vi "Pacemaker Final.vi"() -> ()   [LabVIEW 2018]
panel:
  out "Filtered ECG + Pacemaker Impulses":cluster{"Y":dbl[], dbl[]}[](graph)
  in  "Spreadsheet Path (.csv)":path
  out "ECG Data":dbl[](array[numeric])
  out "Original ECG":waveform(dbl)(graph)
  out "Time Data":dbl
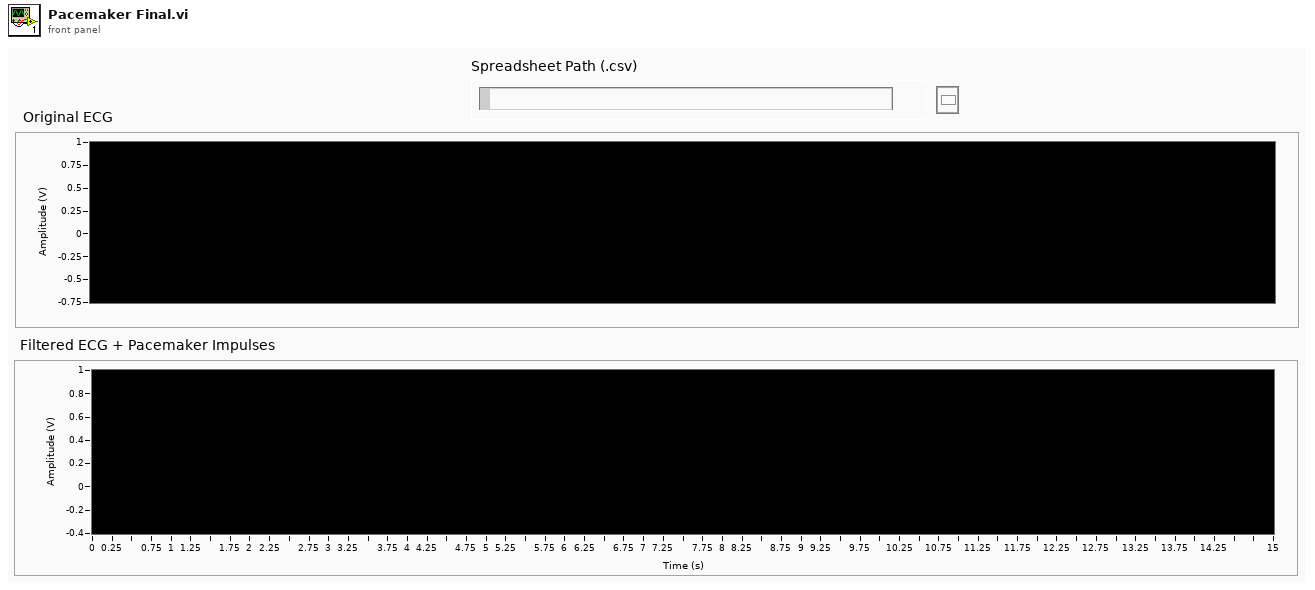
[diagram p1: front panel]
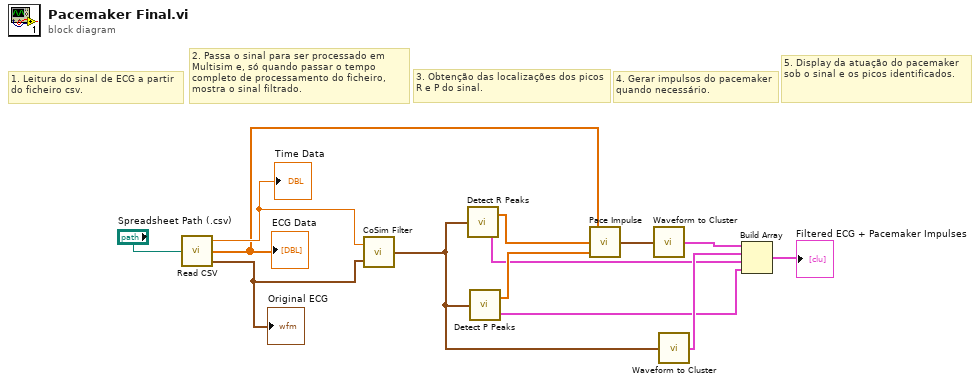
[diagram p0: block diagram]
diagram:
  # "4. Gerar impulsos do pacemaker quando necessário."
  # "3. Obtenção das localizações dos picos R e P do sinal."
  # "5. Display da atuação do pacemaker sob o sinal e os picos identificados."
  # "1. Leitura do sinal de ECG a partir do ficheiro csv."
  # "2. Passa o sinal para ser processado em Multisim e, só quando passar o tempo completo de processamento do ficheiro, mostra o sinal filtrado."
  n1 = call "Read CSV.vi"("file path (dialog if empty)"="Spreadsheet Path (.csv)") -> ("Time Data"=w12:dbl, "ECG Data"=w11:dbl[], "Original ECG"=w10:waveform(dbl))
  "ECG Data" <- w11
  "Original ECG" <- w10
  "Time Data" <- w12
  n2 = call "CoSim Filter.vi"("Original ECG"=w10, "Time Data"=w12) -> ("Filtered ECG"=w6:waveform(dbl))
  n3 = call "Detect R Peaks.vi"("Filtered ECG"=w6) -> ("R-Wave Locations (s)"=w8:dbl[], "Coordinates"=w2:cluster{dbl[], dbl[]})
  n4 = call "Detect P Peaks.vi"("Filtered ECG"=w6) -> ("P-Waves Locations (s)"=w7:dbl[], "Coordinates"=w1:cluster{dbl[], dbl[]})
  n5 = call "Pace Impulse.vi"("P-Waves Locations (s)"=w7, "R-Wave Locations (s)"=w8, "ECG Data"=w11) -> ("Impulses"=w9:waveform(dbl))
  n6 = call "Waveform to Cluster.vi"("Waveform"=w9) -> ("Clustered  Wave"=w4:cluster{"Y":dbl[], dbl[]})
  n7 = call "Waveform to Cluster.vi"("Waveform"=w6) -> ("Clustered  Wave"=w3:cluster{"Y":dbl[], dbl[]})
  n8 = Build Array(w4, w3, w2, w1) -> (→"Filtered ECG + Pacemaker Impulses":cluster{"Y":dbl[], dbl[]}[])
